vi "Confirm Sub-Block.vi"(8 "error in":errorcluster, 11 "Block Upload Sub-Block Transfer in":refnum<class "Block Upload Sub-Block Transfer.lvclass">) -> (0 "error out":errorcluster, 3 "Block Upload Sub-Block Transfer out":refnum<class "Block Upload Sub-Block Transfer.lvclass">)   [LabVIEW 2020, in "CANopen.lvlib" / "SDO Manager.lvlib" / "Block Upload Sub-Block Transfer.lvclass"]
uses:
  Block Upload Sub-Block Transfer.lvclass
  D:/git/CANopen-LabVIEW/source/SDO Manager/SDO Manager/SDO Transfer/SDO Transfer.lvclass
  D:/git/CANopen-LabVIEW/source/SDO Manager/SDO Manager/Block Upload Initiate Transfer/Block Upload Initiate Transfer.lvclass
  SDO Transfer/SDO Transfer.lvclass/SDO Transfer.ctl
  Block Upload Sub-Block Transfer.lvclass/Block Upload Sub-Block Transfer.ctl
  Block Upload Initiate Transfer/Block Upload Initiate Transfer.lvclass/Block Upload Initiate Transfer.ctl
  CANopen Message/CANopen Message.lvclass/CANopen Message.ctl
  HAL/Source/Interfaces/ICommunicate/ICommunicate.lvclass
  CANopen Message/CANopen Message.lvclass
  Typedefs/Function Code.ctl
  CANopen.lvlib
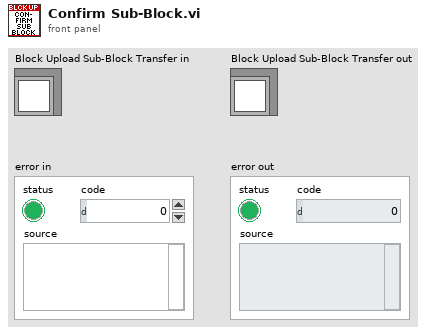
[diagram p1: front panel]
types:
  T1 = typedef "CANopen.lvlib/Function Code.ctl" = u8
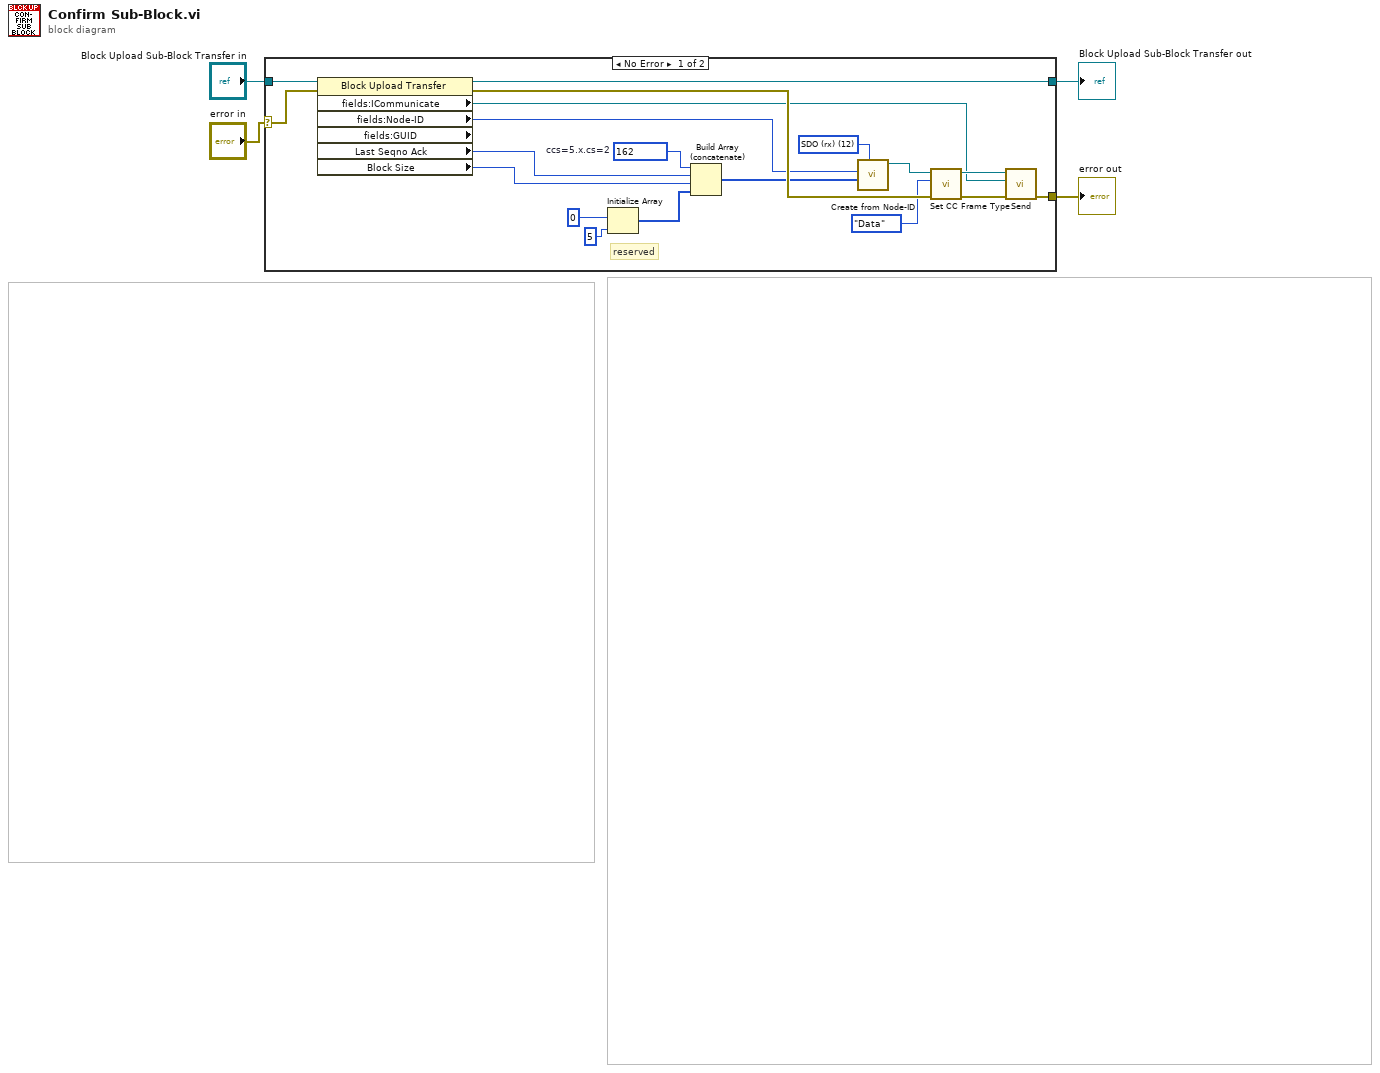
[diagram p0: block diagram]
diagram:
  n1 = case shown="No Error" "error in" {
    selector: "error in" -> [w22 w24]
    tunnel: "Block Upload Sub-Block Transfer in" -> [w21 w25]
    tunnel: [w6 w25] -> w1
    tunnel: [w20 w24] -> w2
    frame No Error {
      w15 = T1 12 items=["NMT"=0, "EMCY/SYNC"=1, "TIME"=2, "PDO1 (tx)"=3, "PDO1 (rx)"=4, "PDO2 (tx)"=5, "PDO2 (rx)"=6, "PDO3 (tx)"=7, "PDO3 (rx)"=8, "PDO4 (tx)"=9, "PDO4 (rx)"=10, "SDO (tx)"=11, "SDO (rx)"=12, "NMT error control"=14] ("Function Code")
      w18 = u8 162  # ccs=5.x.cs=2
      # "reserved"
      n2 = property class="Block Upload Transfer" props=["fields:ICommunicate", "fields:Node-ID", "fields:GUID", "Last Seqno Ack", "Block Size"](reference=w21, error in=w22) -> (reference out=w6:refnum<class "Block Upload Sub-Block Transfer.lvclass">, error out=w23:errorcluster, "fields:ICommunicate"=w7:refnum<class "ICommunicate.lvclass">, "fields:Node-ID"=w19:u8, "Last Seqno Ack"=w5:u8, "Block Size"=w10:u8)  [unwired: 1 out]
      n3 = Initialize Array(u8 0, 5 ("y")) -> (w9:u8[])
      n4 = Build Array (concatenate)(w18, w5, w10, w9) -> (w16:u8[])
      n5 = call "Create from Node-ID.vi"("Function Code"=w15, "Data"=w16, "Node-ID"=w19) -> ("CANopen Message"=w14:refnum<class "CANopen Message.lvclass">)  [unwired: 8 in]
      n6 = call "Set CC Frame Type.vi"("error in"=w23, "CC Frame Type"=enum8{"Data", "Remote", "Error", "Overload"}."Data", "CANopen Message in"=w14) -> ("error out"=w13:errorcluster, "CANopen Message out"=w12:refnum<class "CANopen Message.lvclass">)  [unwired: 7 in]
      n7 = call "Send.vi"("error in"=w13, "ICommunicate"=w7, "CANopen Message in"=w12) -> ("error out"=w20:errorcluster)  [unwired: 7 in, 1 out]
    }
    frame Error {
    }
  }
  "Block Upload Sub-Block Transfer out" <- w1
  "error out" <- w2
